vi "Cleanup.vi"(8 "error in (no error)":errorcluster, 11 "CDebugInfo in":refnum<class "CDebugInfo.lvclass">) -> (0 "error out":errorcluster, 3 "CDebugInfo out":refnum<class "CDebugInfo.lvclass">)   [LabVIEW 2020, in "DependencyInspection.lvlib" / "CDebugInfo.lvclass"]
uses:
  CDebugInfo.lvclass
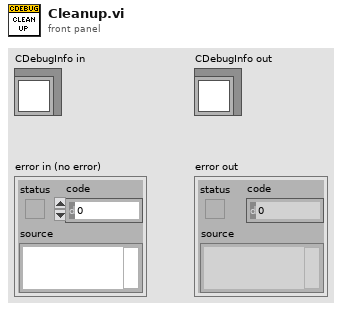
[diagram p1: front panel]
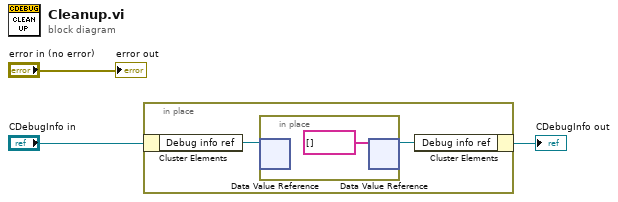
[diagram p0: block diagram]
diagram:
  n1 = in-place {
    n2 = in-place-cluster #1("CDebugInfo in") -> ("Debug info ref"=w5:refnum<data-value>)
    n3 = in-place {
      n4 = in-place-dvr #2(w5) -> ()  [unwired: 2 out]
      n5 = in-place-dvr #2(string[] [] ("data value")) -> (w4:refnum<data-value>)  [unwired: 1 out]
    }
    n6 = in-place-cluster #1("Debug info ref"=w4) -> (→"CDebugInfo out":refnum<class "CDebugInfo.lvclass">)
  }
  "error out" <- "error in (no error)"
